vi "Init Waveform Log.vi"(7 "Waveforms":T1[](array[typedef]), 8 "error in (no error)":errorcluster, 11 "Waveform Log Info":T4 {"Node ID" format="%.0x"; "TDMS Error Code"."Data Ref" format="%.0x"; "Missed Samples"."Data Ref" format="%.0x"; "File Status"."Data Ref" format="%.0x"; "Start New File"."Data Ref" format="%.0x"; "Logging Enabled"."Data Ref" format="%.0x"; "Stop Trigger"."Node Data Ref" format="%.0x"; "Stop Trigger"."Node ID" format="%.0x"; "Start Trigger"."Node Data Ref" format="%.0x"; "Start Trigger"."Node ID" format="%.0x"}) -> (0 "error out":errorcluster, 3 "Waveform Log out":refnum<class "Waveform Log.lvclass">)   [LabVIEW 2015, in "Waveform Log.lvclass"]
uses:
  Waveform Log.lvclass
  Engine/Types/Inline Waveform Log Info.ctl
  Log File Specifications/Waveform TDMS Log File Specification/Waveform TDMS Log File Specification.lvclass
  Triggers/Trigger/Trigger.lvclass
  <vilib>/NI Veristand/Custom Device API/Custom Device Item Ref.ctl
  Engine/Types/Inline Log Waveform.ctl
  Engine/Types/Trigger Settings.ctl
  Engine/Types/Log Status.ctl
  Engine/Types/Channel.ctl
  <vilib>/NI Veristand/Custom Device API/Data Reference.ctl
  Log Waveform.ctl
  Buffer/Waveform Buffer/Waveform Buffer.lvclass
  Waveform Information.ctl
  Waveform Data Type.ctl
  Waveform Log.lvclass/Waveform Log.ctl
  Engine/Waveform Data Logger Engine.lvlib
  <vilib>/NI Veristand/Custom Device API/Custom Device API.lvlib
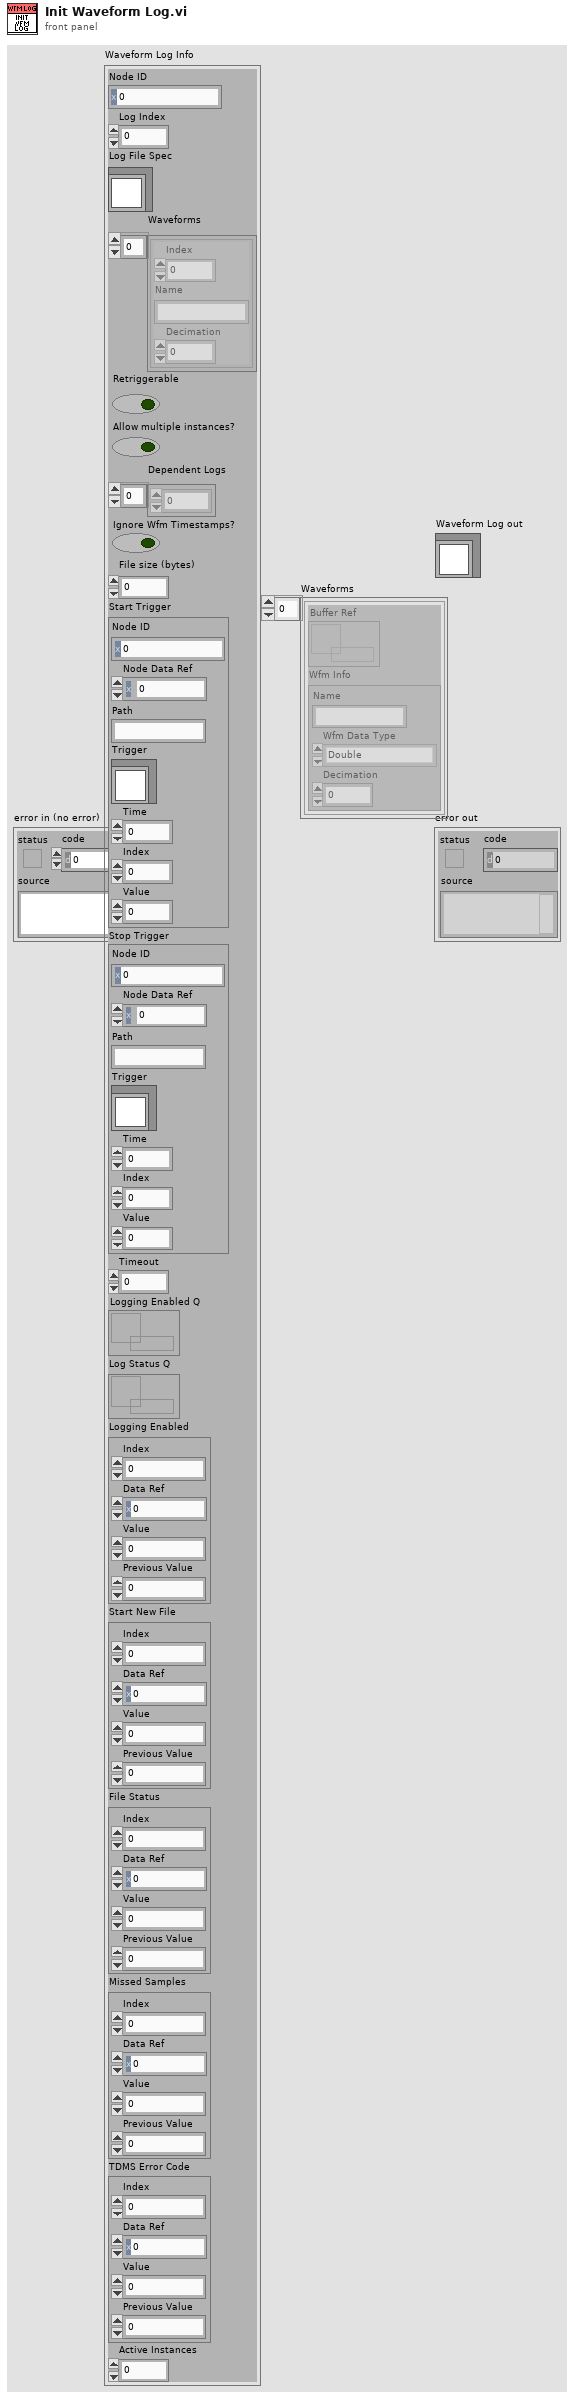
[diagram p1: front panel]
types:
  T1 = typedef "Waveform Log.lvclass/Log Waveform.ctl" = cluster{"Buffer Ref":refnum<data-value>, "Wfm Info":T2}
  T2 = typedef "Waveform Log.lvclass/Waveform Information.ctl" = cluster{"Name":string, "Wfm Data Type":T3, "Decimation":u32}
  T3 = typedef "Waveform Log.lvclass/Waveform Data Type.ctl" = enum16{"Double", "ComplexDouble"}
  T4 = typedef "Waveform Data Logger Engine.lvlib/Inline Waveform Log Info.ctl" = cluster{"Node ID":T5, "Log Index":i32, "Log File Spec":refnum<class "Waveform TDMS Log File Specification.lvclass">, "Waveforms":T6[], "Retriggerable":bool, "Allow multiple instances?":bool, "Dependent Logs":i32[], "Ignore Wfm Timestamps?":bool, "File size (bytes)":i64, "Start Trigger":T7, "Stop Trigger":T7, "Timeout":dbl, "Logging Enabled Q":refnum<queue>, "Log Status Q":refnum<queue>, "Logging Enabled":T8, "Start New File":T8, "File Status":T8, "Missed Samples":T8, "TDMS Error Code":T8, "Active Instances":i32}
  T5 = typedef "Custom Device API.lvlib/Custom Device Item Ref.ctl" = u64
  T6 = typedef "Waveform Data Logger Engine.lvlib/Inline Log Waveform.ctl" = cluster{"Index":i32, "Name":string, "Decimation":u32}
  T7 = typedef "Waveform Data Logger Engine.lvlib/Trigger Settings.ctl" = cluster{"Node ID":T5, "Node Data Ref":i32, "Path":string, "Trigger":refnum<class "Trigger.lvclass">, "Time":dbl, "Index":i32, "Value":dbl}
  T8 = typedef "Waveform Data Logger Engine.lvlib/Channel.ctl" = cluster{"Index":i32, "Data Ref":T9, "Value":dbl, "Previous Value":dbl}
  T9 = typedef "Custom Device API.lvlib/Data Reference.ctl" = i32
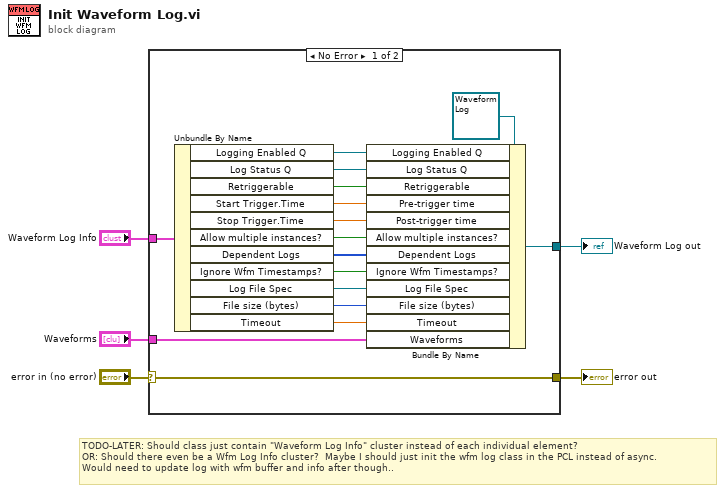
[diagram p0: block diagram]
diagram:
  # "TODO-LATER: Should class just contain \"Waveform Log Info\" cluster instead of each individual element?\nOR: Should there even be a Wfm Log Info cluster?  Maybe I should just init the wfm log class in the PCL instead of async.\nWould need to update log with wfm buffer and info after though.."
  n1 = case shown="No Error" "error in (no error)" {
    selector: "error in (no error)" -> [w21 w22]
    tunnel: [w21 w22] -> w4
    tunnel: [w20 _] -> w3
    tunnel: "Waveform Log Info" -> [w19 _]
    tunnel: "Waveforms" -> [w10 _]
    frame No Error {
      n2 = Unbundle By Name(w19) -> ("Logging Enabled Q"=w7:refnum<queue>, "Log Status Q"=w6:refnum<queue>, "Retriggerable"=w18:bool, "Start Trigger.Time"=w17:dbl, "Stop Trigger.Time"=w16:dbl, "Allow multiple instances?"=w15:bool, "Dependent Logs"=w14:i32[], "Ignore Wfm Timestamps?"=w13:bool, "Log File Spec"=w12:refnum<class "Waveform TDMS Log File Specification.lvclass">, "File size (bytes)"=w11:i64, "Timeout"=w8:dbl)
      n3 = Bundle By Name(cluster=refnum<class "Waveform Log.lvclass"> refnum ("Waveform Log in"), "Logging Enabled Q"=w7, "Log Status Q"=w6, "Retriggerable"=w18, "Pre-trigger time"=w17, "Post-trigger time"=w16, "Allow multiple instances?"=w15, "Dependent Logs"=w14, "Ignore Wfm Timestamps?"=w13, "Log File Spec"=w12, "File size (bytes)"=w11, "Timeout"=w8, "Waveforms"=w10) -> (w20:refnum<class "Waveform Log.lvclass">)
    }
    frame Error {
    }
  }
  "error out" <- w4
  "Waveform Log out" <- w3
